vi "setupLogging.vi"(8 "error in (no error)":errorcluster, 11 "Xcite in":refnum<class "Xcite.lvclass">) -> (0 "error out":errorcluster, 3 "Xcite out":refnum<class "Xcite.lvclass">)   [LabVIEW 2019, in "Xcite.lvclass"]
doc: "Switches on the XCite device output."
uses:
  Xcite.lvclass
  etc.xcite/XCite.lvlib
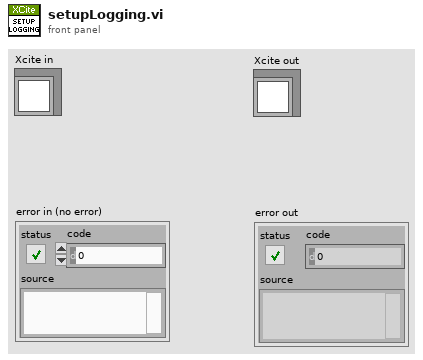
[diagram p1: front panel]
types:
  T1 = enum16{"open", "replace", "create", "open or create", "replace or create", "replace or create with confirmation"}
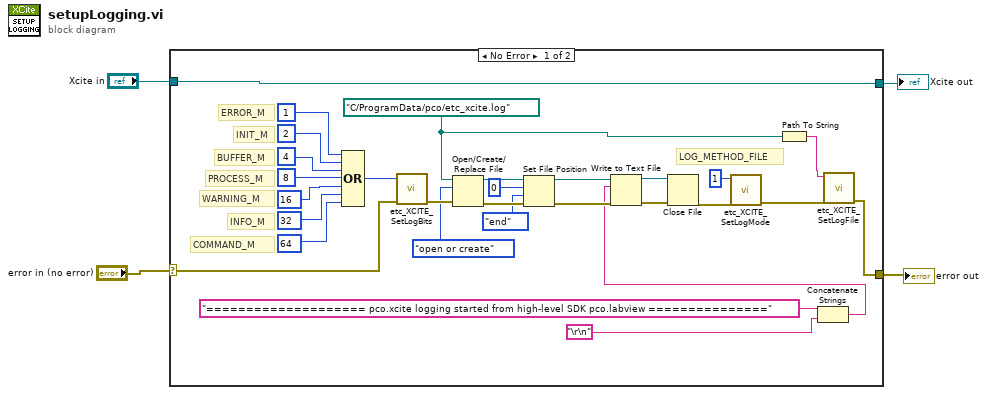
[diagram p0: block diagram]
diagram:
  n1 = case shown="No Error" "error in (no error)" {
    selector: "error in (no error)" -> [w24 w35]
    tunnel: [w16 w35] -> w3
    tunnel: "Xcite in" -> [w33 w34]
    tunnel: [w33 w34] -> w1
    frame No Error {
      w17 = path "C:/ProgramData/pco/etc_xcite.log" ("file path (use dialog)")
      # "LOG_METHOD_FILE"
      # "COMMAND_M"
      # "BUFFER_M"
      # "INFO_M"
      # "WARNING_M"
      # "PROCESS_M"
      # "INIT_M"
      # "ERROR_M"
      n2 = Compound Arithmetic op=OR(u32 1, u32 2, u32 4, u32 8, u32 16, u32 32, u32 64) -> (w25:u32)
      n3 = call "etc_XCITE_SetLogBits.vi"("error in (no error)"=w24, "bits"=w25) -> ("error out"=w22:errorcluster)  [unwired: 9 in]
      n4 = Open/Create/Replace File(file path (use dialog)=w17, error in=w22, operation (0:open)=T1."open or create") -> (refnum out=w12:refnum<file>, error out=w13:errorcluster)  [unwired: 3 in, 1 out]
      n5 = Set File Position(offset (in bytes) (0)=i64 0, refnum=w12, from (0:start)=enum16{"start", "end", "current"}."end", error in=w13) -> (refnum out=w10:refnum<file>, error out=w9:errorcluster)
      n6 = Path To String(path=w17) -> (string=w18:string)
      n7 = Concatenate Strings("==================== pco.xcite logging started from high-level SDK pco.labview ===============" ("text"), "\r\n") -> (w5:string)
      n8 = Write to Text File(file (use dialog)=w10, text=w5, error in=w9) -> (refnum out=w14:refnum<file>, error out=w15:errorcluster)  [unwired: 1 in, 1 out]
      n9 = Close File(refnum=w14, error in=w15) -> (error out=w20:errorcluster)  [unwired: 1 out]
      n10 = call "etc_XCITE_SetLogMode.vi"("error in (no error)"=w20, "mode"=1) -> ("error out"=w19:errorcluster)  [unwired: 9 in]
      n11 = call "etc_XCITE_SetLogFile.vi"("error in (no error)"=w19, "name"=w18) -> ("error out"=w16:errorcluster)  [unwired: 9 in]
    }
    frame Error {
    }
  }
  "Xcite out" <- w1
  "error out" <- w3
